vi "Error.Merge Errors.vi"(1 "First(F)/MergeAll(T)":bool=TRUE, 3 "Errors":errorcluster[](array[cluster])) -> (0 "error out":errorcluster)   [LabVIEW 2018]
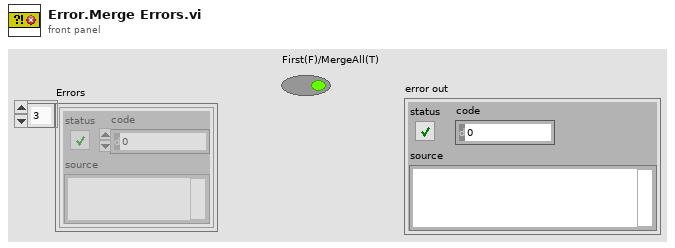
[diagram p1: front panel]
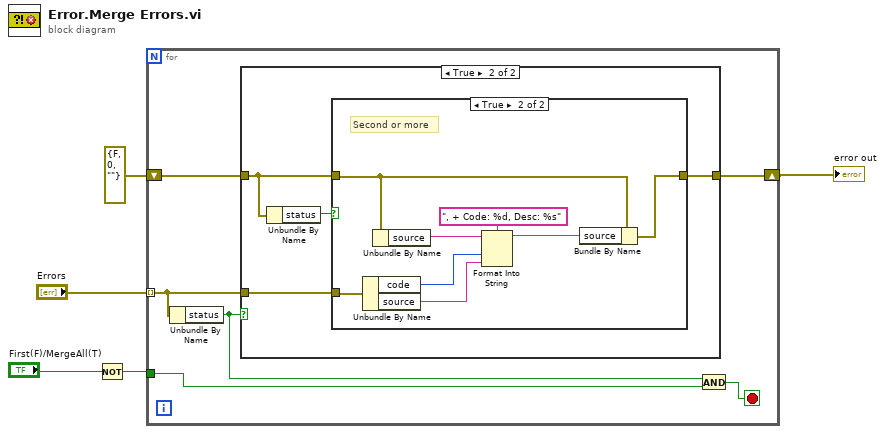
[diagram p0: block diagram]
diagram:
  n1 = Not(x="First(F)/MergeAll(T)") -> (.not. x?=w2:bool)
  n2 = for {
    tunnel: "Errors" -> [w6] mode=indexing
    tunnel: w2 -> [w10]
    shift-right: [w7] -> w3
    shift-left: errorcluster {"status"=FALSE, "code"=0, "source"=""} ("error constant") -> [w8]
    stop <- w11 stop-if-true
    n3 = Unbundle By Name(w6) -> ("status"=w9:bool)
    n4 = case shown="True" w9 {
      tunnel: w8 -> [w12 w15]
      tunnel: [w12 w14] -> w7
      tunnel: w6 -> [_ w13]
      frame False {
      }
      frame True {
        n5 = Unbundle By Name(w15) -> ("status"=w16:bool)
        n6 = case shown="True" w16 {
          tunnel: w15 -> [_ w20]
          tunnel: [w17 w18] -> w14
          tunnel: w13 -> [w17 w25]
          frame False {
            # "First Error"
          }
          frame True {
            # "Second or more"
            n7 = Unbundle By Name(w25) -> ("code"=w22:i32, "source"=w21:string)
            n8 = Unbundle By Name(w20) -> ("source"=w24:string)
            n9 = Format Into String(format string=", + Code: %d, Desc: %s", initial string=w24, w22, w21) -> (resulting string=w19:string)  [unwired: 1 in, 1 out]
            n10 = Bundle By Name(cluster=w20, "source"=w19) -> (w18:errorcluster)
          }
        }
      }
    }
    n11 = And(x=w9, y=w10) -> (x .and. y?=w11:bool)
  }
  "error out" <- w3
